vi "Write ClientNumber.vi"(8 "error in (no error)":errorcluster, 10 "ClientNumber":u16, 11 "ServerListener in":refnum<class "ServerListener.lvclass">) -> (0 "error out":errorcluster, 3 "ServerListener out":refnum<class "ServerListener.lvclass">)   [LabVIEW 2026, in "ServerListener.lvlib" / "ServerListener.lvclass"]
uses:
  ServerListener.lvclass
  ServerListener.lvclass/ServerListener.ctl
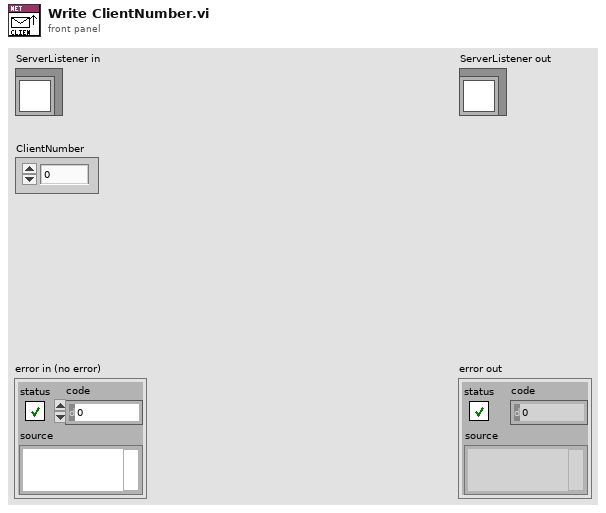
[diagram p1: front panel]
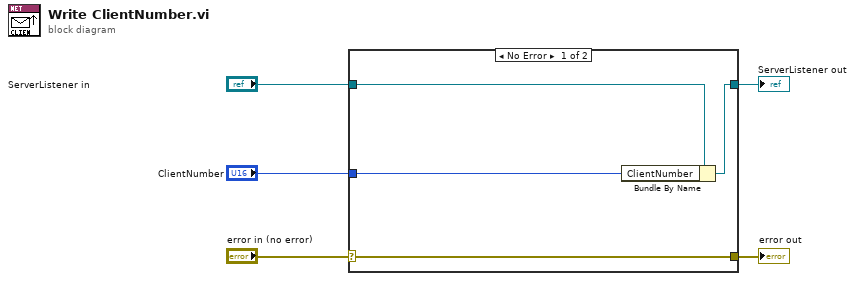
[diagram p0: block diagram]
diagram:
  n1 = case shown="No Error" "error in (no error)" {
    selector: "error in (no error)" -> [w9 w10]
    tunnel: [w9 w10] -> w4
    tunnel: [w7 w11] -> w2
    tunnel: "ServerListener in" -> [w8 w11]
    tunnel: "ClientNumber" -> [w6 _]
    frame No Error {
      n2 = Bundle By Name(cluster=w8, "ClientNumber"=w6) -> (w7:refnum<class "ServerListener.lvclass">)
    }
    frame Error {
    }
  }
  "error out" <- w4
  "ServerListener out" <- w2
